vi "Luanch Logger.vi"(8 "error in (no error)":errorcluster, 9 "Class Name":T2, 10 "Log Level":T1, 11 "Logger Manager":refnum<class "Logger Mananger.lvclass">) -> (0 "error out":errorcluster, 3 "Logger Manager out":refnum<class "Logger Mananger.lvclass">)   [LabVIEW 2020, in "Logging.lvlib" / "Logger Mananger.lvclass"]
uses:
  Logger Mananger.lvclass
  Define/Log Option.ctl
  Define/Log Level.ctl
  C:/Program Files (x86)/National Instruments/LabVIEW 2020/vi.lib/ActorFramework/Actor/Actor.lvclass
  Generic Logger/Generic Logger.lvclass
  Logger Mananger.lvclass/Logger Mananger.ctl
  Generic Logger/Generic Logger.lvclass/Generic Logger.ctl
  <vilib>/ActorFramework/Actor/Actor.lvclass
  Logging.lvlib
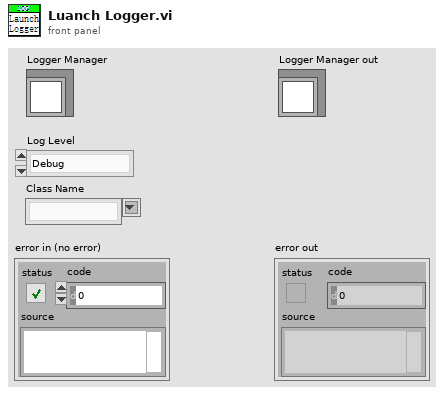
[diagram p1: front panel]
types:
  T1 = typedef "Logging.lvlib/Log Level.ctl" = enum16{"Debug", "Info", "Warn", "Error"}
  T2 = typedef "Logging.lvlib/Log Option.ctl" = string
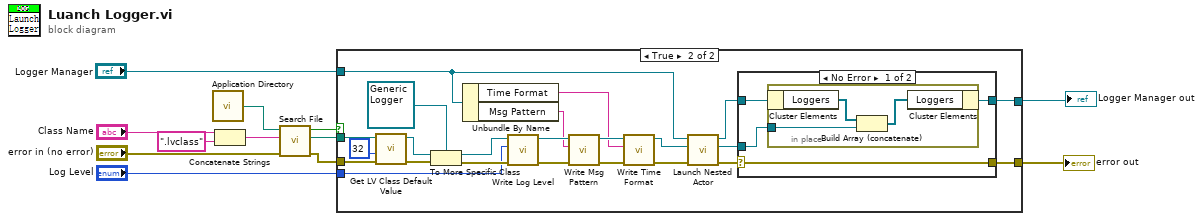
[diagram p0: block diagram]
diagram:
  n1 = call <vilib>:"Application Directory.vi"() -> ("Application Directory"=w12:path)
  n2 = Concatenate Strings("Class Name", ".lvclass" ("string")) -> (w10:string)
  n3 = call "Search File.vi"("error in (no error)"="error in (no error)", "File/Path Name"=w10, "Base Path"=w12) -> ("error out"=w7:errorcluster, "Full path"=w8:path, "Find?"=w9:bool)  [unwired: 6 in]
  n4 = case shown="True" w9 {
    tunnel: w8 -> [_ w37]
    tunnel: w7 -> [w13 w36]
    tunnel: "Log Level" -> [_ w29]
    tunnel: "Logger Manager" -> [w14 w22]
    tunnel: [w14 w17] -> w2
    tunnel: [w13 w18] -> w1
    frame False {
    }
    frame True {
      n5 = call <vilib>:"Get LV Class Default Value.vi"("error in (no error)"=w36, "options"=u32 32, "class path"=w37) -> ("error out"=w33:errorcluster, "object"=w34:refnum<class>)  [unwired: 7 in]
      n6 = To More Specific Class(target class=refnum<class "Generic Logger.lvclass"> refnum ("Logging.lvlib:Generic Logger.lvclass"), reference=w34, error in=w33) -> (specific class reference=w31:refnum<class "Generic Logger.lvclass">, error out=w30:errorcluster)
      n7 = Unbundle By Name(w22) -> ("Time Format"=w21:string, "Msg Pattern"=w20:string)
      n8 = call-dynamic "Write Log Level.vi"("error in (no error)"=w30, "Log Level"=w29, "Logger in"=w31) -> ("error out"=w26:errorcluster, "Logger out"=w28:refnum<class "Generic Logger.lvclass">)  [unwired: 7 in]
      n9 = call "Write Msg Pattern.vi"("error in (no error)"=w26, "Msg Pattern"=w20, "Generic Logger in"=w28) -> ("error out"=w25:errorcluster, "Generic Logger out"=w27:refnum<class "Generic Logger.lvclass">)  [unwired: 7 in]
      n10 = call "Write Time Format.vi"("error in (no error)"=w25, "Time Format"=w21, "Generic Logger in"=w27) -> ("error out"=w23:errorcluster, "Generic Logger out"=w24:refnum<class "Generic Logger.lvclass">)  [unwired: 7 in]
      n11 = call <vilib>:"Launch Nested Actor.vi"("error in (no error)"=w23, "Nested Actor"=w24, "Caller Actor in"=w22) -> ("error out"=w19:errorcluster, "Nested Actor's Enqueuer"=w15:refnum<class "Message Enqueuer.lvclass">, "Caller Actor out"=w16:refnum<class "Logger Mananger.lvclass">)  [unwired: 6 in]
      n12 = case shown="No Error" w19 {
        selector: w19 -> [w40 w46]
        tunnel: [w41 w45] -> w17
        tunnel: [w40 w46] -> w18
        tunnel: w16 -> [w39 w45]
        tunnel: w15 -> [w38 _]
        frame No Error {
          n13 = in-place {
            in-place-border: w38 -> [w44]
            n14 = in-place-cluster #1(w39) -> ("Loggers"=w43:refnum<class "Message Enqueuer.lvclass">[])
            n15 = Build Array (concatenate)(w43, w44) -> (w42:refnum<class "Message Enqueuer.lvclass">[])
            n16 = in-place-cluster #1("Loggers"=w42) -> (w41:refnum<class "Logger Mananger.lvclass">)
          }
        }
        frame Error {
        }
      }
    }
  }
  "Logger Manager out" <- w2
  "error out" <- w1
